vi "Line Midpoint.vi"(3 "Midpoint":T1 {"Y" format="%.2f"; "X" format="%.2f"}, 8 "error in (no error)":errorcluster, 10 "Point 2":T1 {"Y" format="%.2f"; "X" format="%.2f"}, 11 "Point 1":T1 {"Y" format="%.2f"; "X" format="%.2f"}) -> (0 "error out":errorcluster)   [LabVIEW 2013]
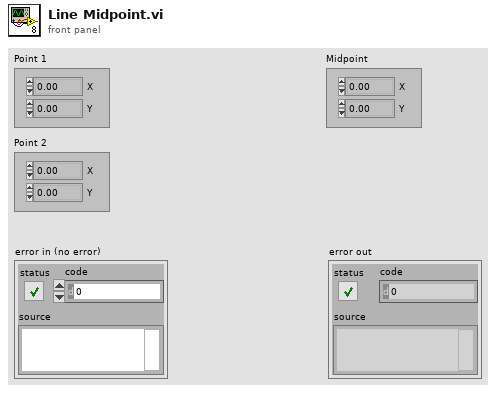
[diagram p1: front panel]
types:
  T1 = typedef "IMAQ Point" = cluster{"X":sgl, "Y":sgl}
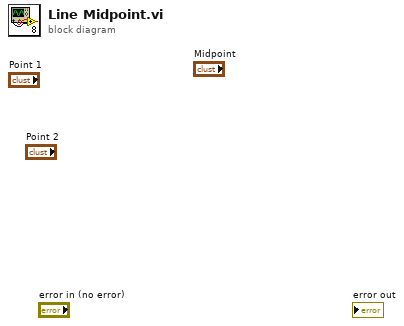
[diagram p0: block diagram]
diagram:
